vi "Init Conf File.vi"(8 "error in":errorcluster, 11 "Test Stand in":refnum<class "Generic Test Stand.lvclass">) -> (0 "error out":errorcluster, 1 "Conf Filename":string, 3 "Test Stand out":refnum<class "Generic Test Stand.lvclass">)   [LabVIEW 2019, in "Generic Test Stand.lvclass"]
uses:
  Generic Test Stand.lvclass
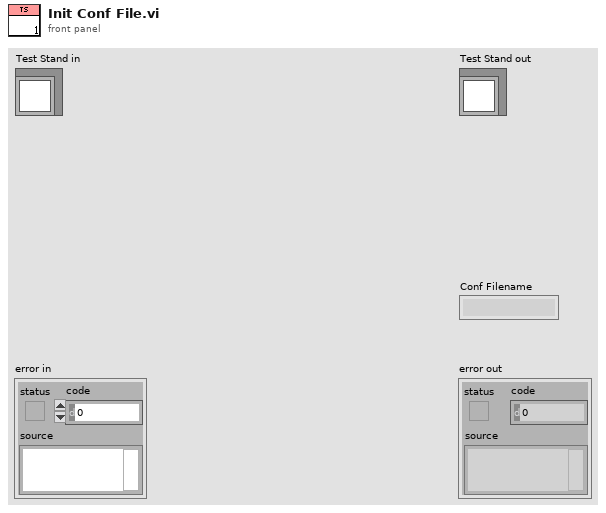
[diagram p1: front panel]
types:
  T1 = enum16{"open", "replace", "create", "open or create", "replace or create", "replace or create with confirmation"}
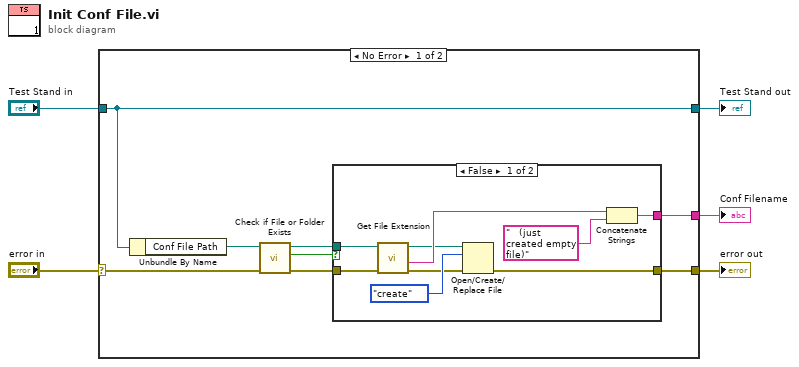
[diagram p0: block diagram]
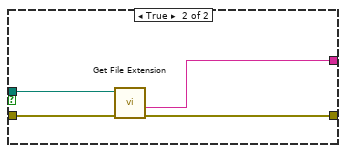
[diagram p2: hidden frame]
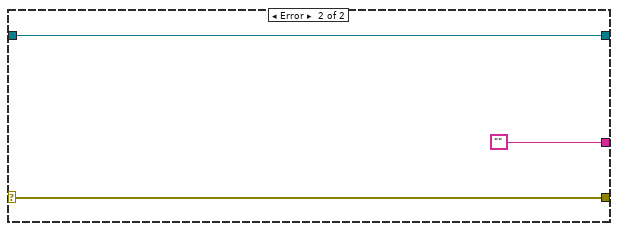
[diagram p3: hidden frame]
diagram:
  n1 = case shown="No Error" "error in" {
    selector: "error in" -> [w8 w29]
    tunnel: [w6 w29] -> w4
    tunnel: [w10 w28] -> w2
    tunnel: "Test Stand in" -> [w10 w28]
    tunnel: [w7 ""] -> w1
    frame No Error {
      n2 = Unbundle By Name(w10) -> ("Conf File Path"=w9:path)
      n3 = call <vilib>:"Check if File or Folder Exists.vi"("error in (no error)"=w8, "path"=w9) -> ("error out"=w11:errorcluster, "file or folder exists?"=w13:bool, "dup path"=w12:path)  [unwired: 7 in]
      n4 = case shown="False" w13 {
        tunnel: w12 -> [w21 w26]
        tunnel: [w18 w25] -> w7
        tunnel: w11 -> [w16 w24]
        tunnel: [w14 w23] -> w6
        frame False {
          n5 = call <vilib>:"Get File Extension.vi"("error in (no error)"=w16, "file"=w21) -> ("error out"=w15:errorcluster, "filename without extension"=w19:string, "dup file"=w17:path)  [unwired: 5 in, 2 out]
          n6 = Open/Create/Replace File(file path (use dialog)=w17, error in=w15, operation (0:open)=T1."create") -> (error out=w14:errorcluster)  [unwired: 3 in, 2 out]
          n7 = Concatenate Strings(w19, "   (just created empty file)" ("string")) -> (w18:string)
        }
        frame True {
          n8 = call <vilib>:"Get File Extension.vi"("error in (no error)"=w24, "file"=w26) -> ("error out"=w23:errorcluster, "filename without extension"=w25:string)  [unwired: 5 in, 3 out]
        }
      }
    }
    frame Error {
    }
  }
  "error out" <- w4
  "Test Stand out" <- w2
  "Conf Filename" <- w1
